vi "7.7.3-UDP-OCU_to_Forbrain-Server.vi"() -> ()   [LabVIEW 2010]
doc: "Creates a named service and listens on the first available port. Whenever a client connects to the service, it responds with a message containing joystick data. The VI can be stopped using the STOP button."
uses:
  6-OCU Neurons/AutoModeControls.ctl
  7.0-Global.vi
panel:
  out "7.7.1 AutoModeDatums":T1
  out "data out":string
  out "error out":errorcluster
  in  "error in":errorcluster
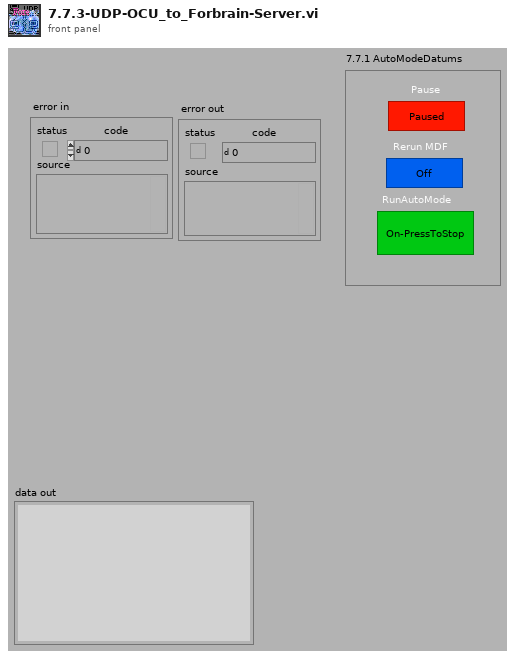
[diagram p1: front panel]
types:
  T1 = typedef "AutoModeControls.ctl" = cluster{"RunAutoMode":bool, "Rerun MDF":bool, "Pause":bool}
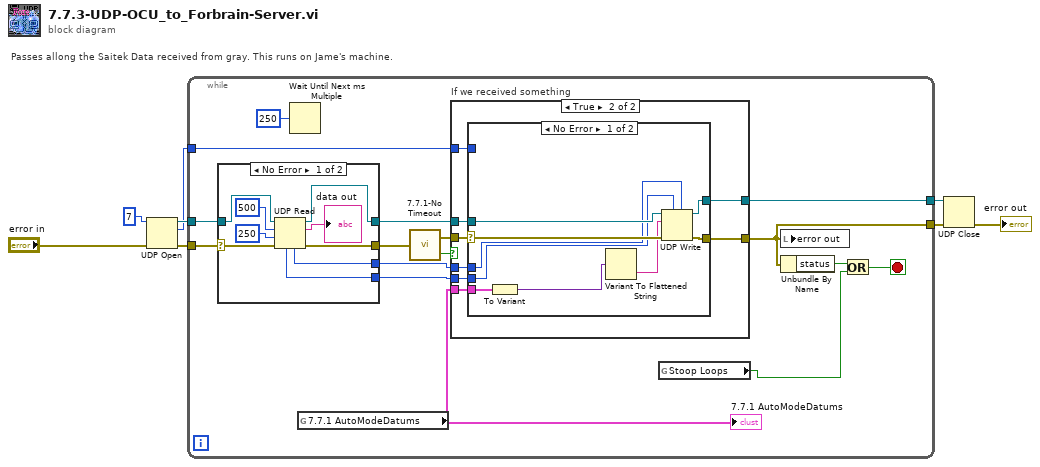
[diagram p0: block diagram]
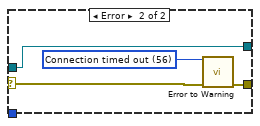
[diagram p3: hidden frame]
diagram:
  # "Passes allong the Saitek Data received from gray. This runs on Jame's machine."
  n1 = UDP Open(8:"error in", 11:u16 7) -> (port=w6:refnum<k16>, 0:w5:errorcluster, 2:w1:u16)  [unwired: 3 in]
  n2 = while {
    tunnel: [w13] -> w3
    tunnel: w6 -> [w24]
    tunnel: w5 -> [w21]
    tunnel: [w22] -> w4
    tunnel: w1 -> [w18]
    stop <- w16 stop-if-true
    n3 = case shown="No Error" w21 {
      selector: w21 -> [w54 w57]
      tunnel: w24 -> [w56 w58]
      tunnel: [w53 w58] -> w23
      tunnel: [w52 w57] -> w12
      tunnel: [w50 _] -> w19
      tunnel: [w51 _] -> w20
      frame No Error {
        n4 = UDP Read(connection ID=w56, max size (548)=500, timeout ms (25000)=250, 8:w54) -> (data out=→"data out":string, error out=w52:errorcluster, 3:w53:refnum<k16>, 4:w50:u16, 6:w51:u32)
      }
      frame Error {
      }
    }
    n5 = Wait Until Next ms Multiple(millisecond multiple=u32 250) -> ()  [unwired: 1 out]
    n6 = global read "7.0-Global.vi" "7.7.1 AutoModeDatums"() -> (w11:T1)
    "7.7.1 AutoModeDatums" <- w11
    n7 = call "7.7.1-No Timeout.vi"("error in (no error)"=w12) -> ("No Timeout"=w14:bool, "error out"=w15:errorcluster)
    n8 = case "If we received something" shown="True" w14 {
      tunnel: w23 -> [w25 w34]
      tunnel: [w25 w33] -> w22
      tunnel: w20 -> [_ w32]
      tunnel: w19 -> [_ w31]
      tunnel: w18 -> [_ w30]
      tunnel: [w26 w29] -> w13
      tunnel: w15 -> [w26 w28]
      tunnel: w11 -> [_ w27]
      frame False {
      }
      frame True {
        n9 = case shown="No Error" w28 {
          selector: w28 -> [w43 w45]
          tunnel: w34 -> [w40 w47]
          tunnel: [w42 w44] -> w29
          tunnel: [w41 w47] -> w33
          tunnel: w32 -> [w38 _]
          tunnel: w31 -> [w39 _]
          tunnel: w30 -> [_ _]
          tunnel: w27 -> [w35 _]
          frame No Error {
            n10 = To Variant(anything=w35) -> (Variant=w37:variant)
            n11 = Variant To Flattened String(Variant=w37) -> (data string=w36:string)  [unwired: 1 out]
            n12 = UDP Write(address=w38, port or service name=w39, connection ID=w40, data in=w36, 8:w43) -> (error out=w42:errorcluster, 3:w41:refnum<k16>)  [unwired: 1 in]
          }
          frame Error {
            w46 = 56 items=["No Error", "Argument Error", "Memory Full", "Out of Zone", "End of File", "File Already Open", "Generic File IO Error", "File Not Found", "File Permission Error", "Disk Full", "Duplicate Path", "Too Many Files Open", "Not Enabled", "Resource File Not Found", "Cannot Add Resource", "Resource Not Found", "Image Not Found", "Image Memory Error", "Pen Does Not Exist", "Config Bad Type", "Config Token Not Found", "Config Parse Error", "Config Memory Error", "Bad External Code Format", "Bad External Code Offset", "External Code Not Present", "Null Window", "Destroy Window Mixup", "Null Menu", "Print Aborted", "Bad Print Record", "Print Driver Error", "Windows Error During Print", "Memory Error During Print", "Print Dialog Error", "Generic Print Error", "Invalid Device Refnum", "Device Not Found", "Device Parameter Error", "Device Unit Error", "Can't Open Device", "Device Call Aborted", "Generic Error", "Cancelled By User", "Object ID Too Low", "Object ID Too High", "Object Not In Heap", "Unknown Heap", "Bad DefProc ID", "DefProc Not In Table", "Message Out Of Range", "Null Method", "Unknown Message", "Manager Call Not Supported", "Bad address", "Connection In progress", "Connection timed out", "Connection is already in progress", "Network attribute not supported", "Network error", "Address in use", "System out of memory", "Connection aborted", "Connection refused", "Connection is not connected", "Connection is already connected", "Connection closed", "Initialize error (interapplication manager)", "Bad occurrence", "Wait on unbound occurrence handler", "Occurrence queue overflow", "Bad path", "Semaphore not signaled", "Unrecognized type (interapplication manager)"] ("1st Error to Convert")
            n13 = call <vilib>:"Error to Warning.vi"("1st Error to Convert"=w46, "error in"=w45) -> ("warning out"=w44:errorcluster)  [unwired: 13 in]
          }
        }
      }
    }
    n14 = global read "7.0-Global.vi" "Stoop Loops"() -> (w10:bool)
    n15 = local write "error out"(w13) -> ()
    n16 = Unbundle By Name(w13) -> ("status"=w17:bool)
    n17 = Or(x=w17, y=w10) -> (x .or. y?=w16:bool)
  }
  n18 = UDP Close(connection ID=w4, 8:w3) -> (error out=→"error out":errorcluster)  [unwired: 1 out]
